vi "FRAS Calcul CdG.vi"(0 "Tableau X":i32[](array[numeric]), 5 "Tableau Y":i32[](array[numeric]), 7 "Imagette seuillée":i16[][](array[numeric]), 9 "Largeur cote":i32) -> (8 "CdG":sgl[](array[numeric]))   [LabVIEW 2020]
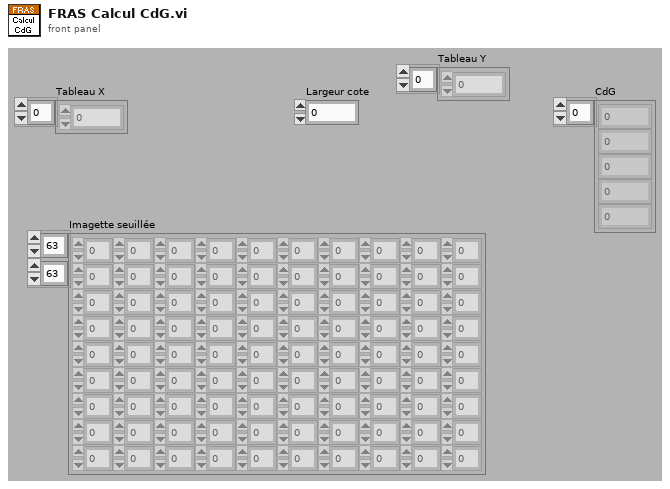
[diagram p1: front panel]
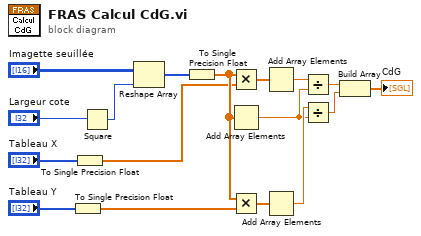
[diagram p0: block diagram]
diagram:
  n1 = To Single Precision Float(number="Tableau Y") -> (single precision float=w1:sgl[])
  n2 = To Single Precision Float(number="Tableau X") -> (single precision float=w2:sgl[])
  n3 = Square(x="Largeur cote") -> (x^2=w17:i32)
  n4 = Reshape Array("Imagette seuillée", w17) -> (w5:i16[])
  n5 = To Single Precision Float(number=w5) -> (single precision float=w3:sgl[])
  n6 = Multiply(x=w3, y=w2) -> (x*y=w12:sgl[])
  n7 = Add Array Elements(numeric array=w3) -> (sum=w8:sgl)
  n8 = Multiply(x=w3, y=w1) -> (x*y=w11:sgl[])
  n9 = Add Array Elements(numeric array=w12) -> (sum=w10:sgl)
  n10 = Add Array Elements(numeric array=w11) -> (sum=w9:sgl)
  n11 = Divide(x=w10, y=w8) -> (x/y=w7:sgl)
  n12 = Divide(x=w9, y=w8) -> (x/y=w6:sgl)
  n13 = Build Array(w7, w6) -> (→"CdG":sgl[])
